vi "Ex1 Image Import.vi"() -> ()   [LabVIEW 2020]
panel:
  out "error out":errorcluster
  in  "Image Type":T1 items=["Grayscale (U8)", "Grayscale (I16)", "Grayscale (SGL)", "Complex (CSG)", "RGB (U32)", "HSL (U32)", "RGB (U64)", "Grayscale (U16)"]
  out "Image":T2(plugin-control)
  in  "File Path":path
  # "EX.1 Image Import"
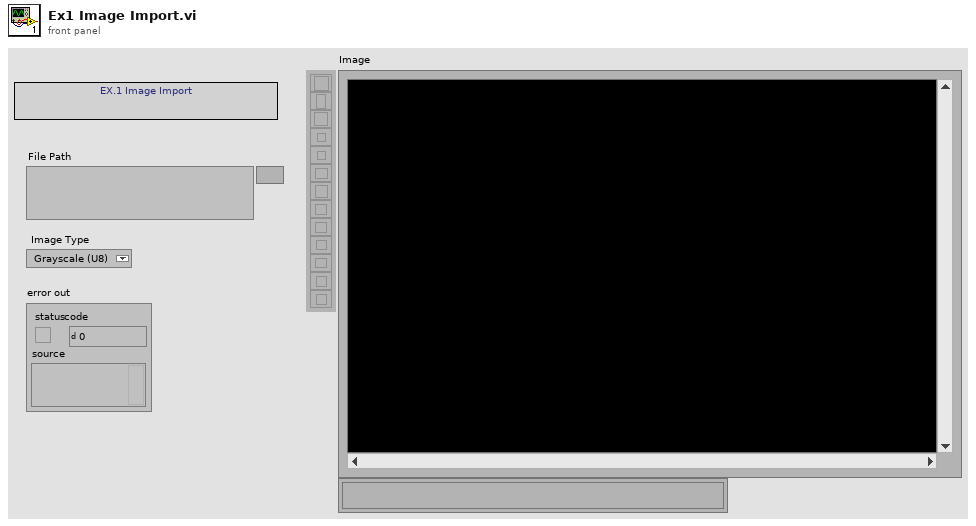
[diagram p1: front panel]
types:
  T1 = typedef "Image Type" = u32
  T2 = typedef "IMAQ Image.ctl" = refnum<image>
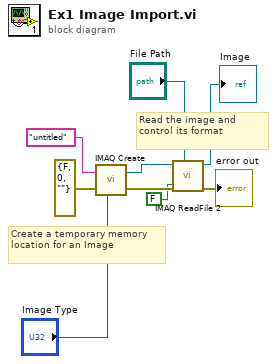
[diagram p0: block diagram]
diagram:
  # "Read the image and control its format"
  # "Create a temporary memory location for an Image"
  n1 = call "IMAQ Create"("Image Name"="untitled", "Image Type"="Image Type", "error in (no error)"=errorcluster {"status"=FALSE, "code"=0, "source"=""}) -> ("New Image"=w7:T2, "error out"=w5:errorcluster)  [unwired: 2 in]
  n2 = call "IMAQ ReadFile 2"("Use File Path Image Type"=FALSE, "File Path"="File Path", "error in (no error)"=w5, "Image"=w7) -> ("error out"=→"error out":errorcluster, "Image Out"=→"Image":T2)  [unwired: 3 in, 3 out]
